vi "Analysis Info Cluster Variables.vi"() -> (0 "Array":string[](array[string]))   [LabVIEW 2022 SP3]
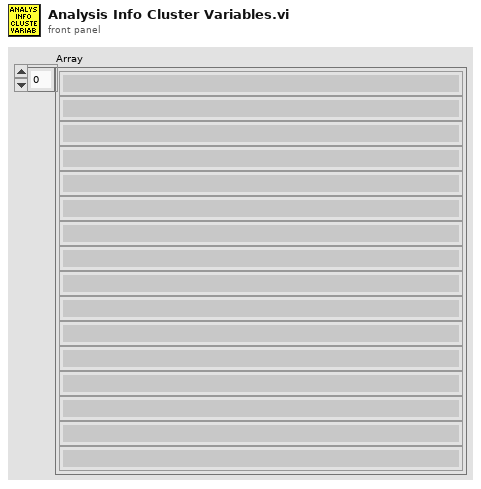
[diagram p1: front panel]
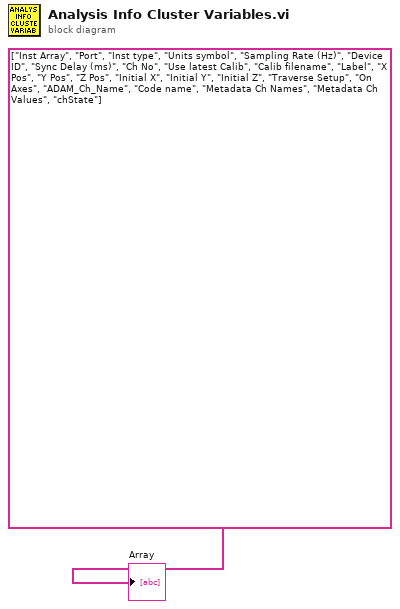
[diagram p0: block diagram]
diagram:
  "Array" <- string[] ["Inst Array", "Port", "Inst type", "Units symbol", "Sampling Rate (Hz)", "Device ID", "Sync Delay (ms)", "Ch No", "Use latest Calib", "Calib filename", "Label", "X Pos", "Y Pos", "Z Pos", "Initial X", "Initial Y", "Initial Z", "Traverse Setup", "On Axes", "ADAM_Ch_Name", "Code name", "Metadata Ch Names", "Metadata Ch Values", "chState"]
